vi "pf_Plot_3D_CoP.vi"(3 "error in (no error)":errorcluster, 4 "Range Map in":sgl[][](array[numeric]), 5 "3D Surface":refnum<k7>(container)) -> (0 "error out":errorcluster)   [LabVIEW 2025, in "Photonfocus_Toolkit.lvlib"]
uses:
  Photonfocus_Toolkit.lvlib
panel:
  in  "IMAQ Session in":refnum<k11>
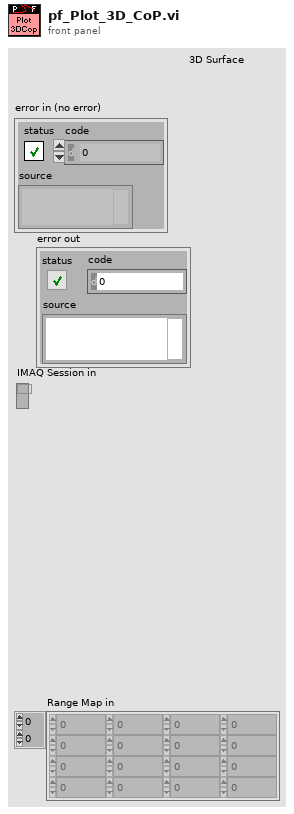
[diagram p1: front panel]
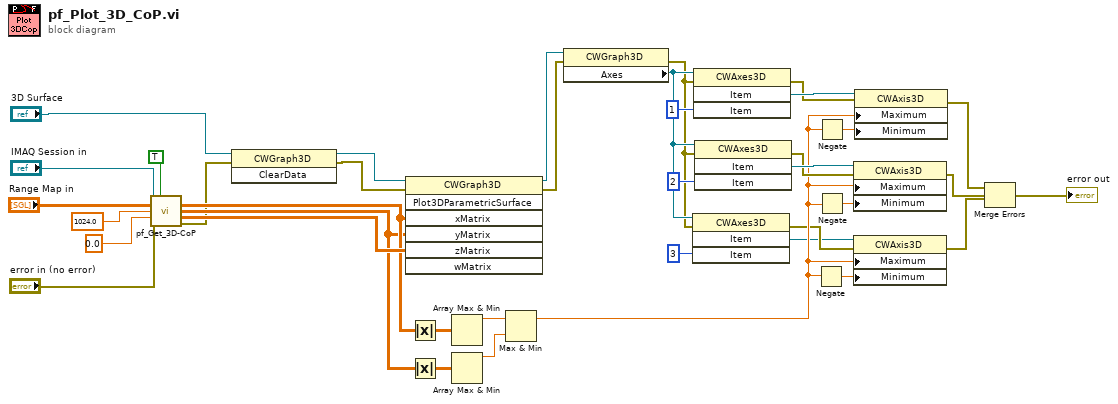
[diagram p0: block diagram]
diagram:
  n1 = call "pf_Get_3D-CoP.vi"("IMAQ Session in"="IMAQ Session in", "Truncate Range"=TRUE, "Range Map in"="Range Map in", "Range Max"=sgl 1024.0, "Range Min"=sgl 0.0, "error in (no error)"="error in (no error)") -> ("X Matrix"=w27:sgl[][], "Y Matrix"=w26:sgl[][], "Z Matrix"=w38:sgl[][], "error out"=w3:errorcluster)  [unwired: 2 in, 4 out]
  n2 = invoke class="CWGraph3D" method="ClearData"(reference="3D Surface", error in=w3) -> (reference out=w5:refnum<k7>, error out=w4:errorcluster)  [unwired: 1 in, 1 out]
  n3 = invoke class="CWGraph3D" method="Plot3DParametricSurface"(reference=w5, error in=w4, "xMatrix"=w27, "yMatrix"=w26, "zMatrix"=w38) -> (reference out=w35:refnum<k7>, error out=w34:errorcluster)  [unwired: 2 in, 5 out]
  n4 = Absolute Value(x=w27) -> (abs(x)=w25:sgl[][])
  n5 = Absolute Value(x=w26) -> (abs(x)=w24:sgl[][])
  n6 = Array Max & Min(array=w25) -> (max value=w23:sgl)  [unwired: 3 out]
  n7 = Array Max & Min(array=w24) -> (max value=w22:sgl)  [unwired: 3 out]
  n8 = Max & Min(x=w23, y=w22) -> (max(x,y)=w15:sgl)  [unwired: 1 out]
  n9 = property class="CWGraph3D"(reference=w35, error in=w34) -> (error out=w12:errorcluster, "Axes"=w17:refnum<k7>)  [unwired: 1 out]
  n10 = invoke class="CWAxes3D" method="Item"(reference=w17, error in=w12, "Item"=3) -> (error out=w11:errorcluster, "Item"=w10:refnum<k7>)  [unwired: 1 in, 2 out]
  n11 = invoke class="CWAxes3D" method="Item"(reference=w17, error in=w12, "Item"=1) -> (error out=w29:errorcluster, "Item"=w32:refnum<k7>)  [unwired: 1 in, 2 out]
  n12 = invoke class="CWAxes3D" method="Item"(reference=w17, error in=w12, "Item"=2) -> (error out=w28:errorcluster, "Item"=w31:refnum<k7>)  [unwired: 1 in, 2 out]
  n13 = Negate(x=w15) -> (-x=w14:sgl)
  n14 = Negate(x=w15) -> (-x=w20:sgl)
  n15 = Negate(x=w15) -> (-x=w21:sgl)
  n16 = property class="CWAxis3D"(reference=w31, error in=w28, "Maximum"=w15, "Minimum"=w21) -> (error out=w18:errorcluster)  [unwired: 1 out]
  n17 = property class="CWAxis3D"(reference=w10, error in=w11, "Maximum"=w15, "Minimum"=w14) -> (error out=w13:errorcluster)  [unwired: 1 out]
  n18 = property class="CWAxis3D"(reference=w32, error in=w29, "Maximum"=w15, "Minimum"=w20) -> (error out=w19:errorcluster)  [unwired: 1 out]
  n19 = Merge Errors(w19, w18, w13) -> (→"error out":errorcluster)
